vi "E4440A_PSA_Marker_Query.vi"(8 "error in (no error)":errorcluster, 10 "Active Marker (1: Marker1)":u16(ring)=1 items=["Marker1"=1, "Marker2"=2, "Marker3"=3, "Marker4"=4], 11 "VISA resource name":refnum<visa-resource-name>) -> (0 "error out":errorcluster, 1 "Marker Amplitude":dbl, 2 "Marker Position":dbl, 3 "VISA resource name out":refnum<visa-resource-name>)   [LabVIEW 2015]
doc: "Returns the x-position and amplitude of a specified marker."
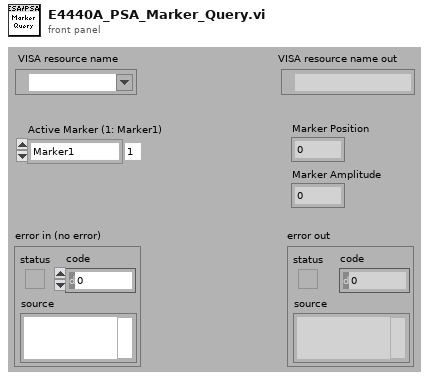
[diagram p1: front panel]
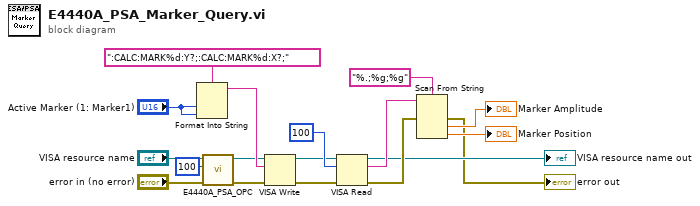
[diagram p0: block diagram]
diagram:
  n1 = Format Into String(format string=":CALC:MARK%d:Y?;:CALC:MARK%d:X?;", "Active Marker (1: Marker1)", "Active Marker (1: Marker1)") -> (resulting string=w16:string)  [unwired: 2 in, 1 out]
  n2 = call "E4440A_PSA_OPC.vi"("error in (no error)"="error in (no error)", "Wait (1000ms)"=u32 100, "VISA resource name"="VISA resource name") -> ("error out"=w4:errorcluster, "VISA resource name out"=w2:refnum<visa-resource-name>)  [unwired: 7 in]
  n3 = VISA Write(VISA resource name=w2, write buffer=w16, error in (no error)=w4) -> (VISA resource name out=w5:refnum<visa-resource-name>, error out=w6:errorcluster)  [unwired: 1 out]
  n4 = VISA Read(VISA resource name=w5, byte count=u32 100, error in (no error)=w6) -> (VISA resource name out=→"VISA resource name out":refnum<visa-resource-name>, read buffer=w13:string, error out=w14:errorcluster)  [unwired: 1 out]
  n5 = Scan From String(format string="%.;%g;%g", input string=w13, error in=w14) -> (error out=→"error out":errorcluster, output 1=→"Marker Amplitude":dbl, output 2=→"Marker Position":dbl)  [unwired: 3 in, 2 out]
